vi "PQsetnonblocking.vi"(8 "error in (no error)":errorcluster, 10 "arg":i64, 11 "conn":u64) -> (0 "error out":errorcluster, 2 "PQsetnonblocking":i64, 3 "conn_out":u64)   [LabVIEW 2019, in "libpqlv64.lvlib"]
doc: "PQsetnonblocking\n\n Sets the nonblocking status of the connection.\n\n int PQsetnonblocking(PGconn *conn, int arg);\n\n Sets the state of the connection to nonblocking if arg is 1, or blocking if arg is 0. Returns 0 if OK, -1 if error.\n\n In the nonblocking state, calls to PQsendQuery, PQputline, PQputnbytes, and PQendcopy will not block but instead return an error if they need to be called again.\n\n Note that PQexec does not honor nonblocking mode; if it is called, it will act in blocking fashion anyway. \nhttp://www.postgresql.org/docs/8.3/static/libpq-async.html"
uses:
  libpqlv64.lvlib
  libpq.dll
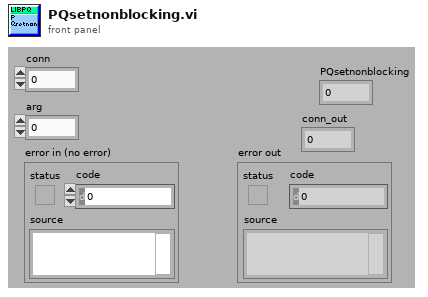
[diagram p1: front panel]
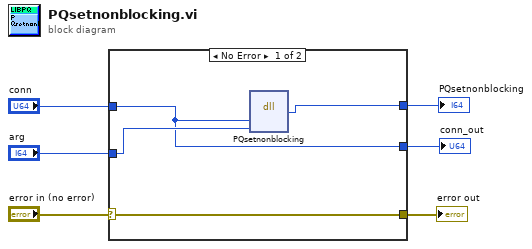
[diagram p0: block diagram]
diagram:
  n1 = case shown="No Error" "error in (no error)" {
    selector: "error in (no error)" -> [w10 w12]
    tunnel: [w10 w12] -> w5
    tunnel: [w9 _] -> w4
    tunnel: "arg" -> [w8 _]
    tunnel: "conn" -> [w7 w11]
    tunnel: [w7 w11] -> w1
    frame No Error {
      n2 = dll-call lib="libpq.*" fn="PQsetnonblocking"("conn"=w7, "arg"=w8) -> ("PQsetnonblocking"=w9:i64)  [unwired: 5 in, 2 out]
    }
    frame Error {
    }
  }
  "PQsetnonblocking" <- w4
  "error out" <- w5
  "conn_out" <- w1
